vi "固件升级（包含参数恢复）.vi"() -> (3 "结果字符串":string)   [LabVIEW 2016, in "斯坦道总磷.lvlib"]
uses:
  <vilib>/NI/Progress Bar/Progress Bar.lvlib
  <vilib>/NI/Progress Bar/Controls/Progress Bar Properties.ctl
panel:
  out "固件升级步骤":T1
  # "固件升级步骤：\n1、读取固件状态\n2、读取仪器外设设置\n3、读取仪器试剂容量设置\n4、读取仪器量程参数设置\n5、读取仪器公式\n6、写入仪器固件\n7、写入仪器外设设置\n8、写入仪器试剂容量设置\n9、写入仪器量程参数设置\n10、写入仪器公式\n11、询问是否写入流程"
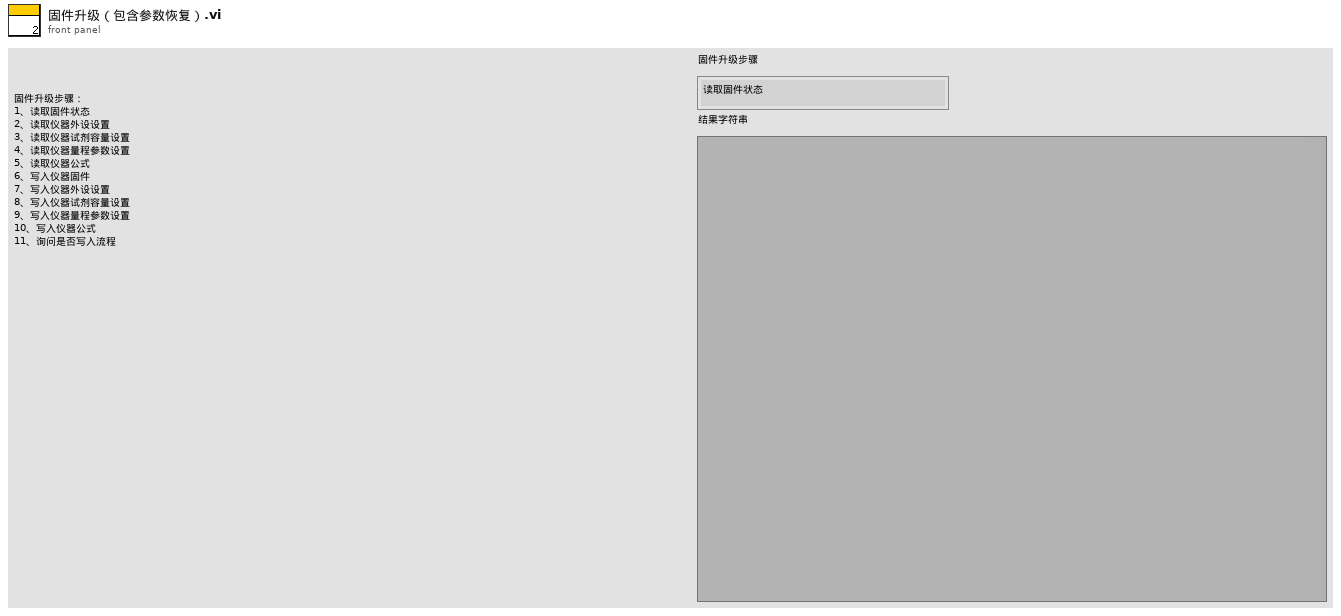
[diagram p1: front panel]
types:
  T1 = typedef "斯坦道总磷.lvlib/固件升级步骤.ctl" = enum16{"读取固件状态", "读取仪器外设设置", "读取仪器试剂容量设置", "读取仪器量程参数设置", "读取仪器公式", "写入仪器固件", "写入仪器外设设置", "写入仪器试剂容量设置", "写入仪器量程参数", "写入仪器公式", "询问是否写入流程", "写入测试流程", "结束"}
  T2 = typedef "Progress Bar.lvlib/Progress Bar Properties.ctl" = cluster{"Background Color":u32, "Installer Title":string, "Title Color":u32, "Action Text":string, "Text Color":u32, "Slider Value":u8, "Bar Color":u32, "Timeout":i32}
  T3 = cluster{"泵类型":u8, "进样速度":u32, "出样速度":u32, "泵阀量":u8, "光谱仪类型":u8, "光谱采样次数":u8, "氙灯次数":u8, "B":u16, "C":u16, "D":u16, "E":u16, "B_COD":u16, "C_COD":u16, "D_COD":u16, "E_COD":u16, "G":u16, "M":u16, "N":u16, "氨氮注射泵控温下限":sgl, "氨氮注射泵控温上限":sgl, "总氮注射泵控温下限":sgl, "总氮注射泵控温上限":sgl, "消解温度下限":sgl, "消解温度上限":sgl, "加热10s限值":sgl, "高温高压阀开阀温度":sgl, "总氮x公式0":u8, "总氮x公式1":sgl, "总氮x公式2":sgl, "总磷浊度稀释系数":sgl, "总磷浊度补偿权重1":sgl, "总磷浊度补偿权重2":sgl, "盐度系数":sgl, "氨氮补偿系数1":sgl, "氨氮补偿系数2":sgl}
  T4 = cluster{"外设配置":cluster{"泵类型":u8, "进样速度":u32, "出样速度":u32, "泵阀量":u8, "光谱仪类型":u8, "光谱采样次数":u8, "氙灯次数":u8, "B":u16, "C":u16, "D":u16, "E":u16, "B_COD":u16, "C_COD":u16, "D_COD":u16, "E_COD":u16, "G":u16, "M":u16, "N":u16, "氨氮注射泵控温下限":sgl, "氨氮注射泵控温上限":sgl, "总氮注射泵控温下限":sgl, "总氮注射泵控温上限":sgl, "消解温度下限":sgl, "消解温度上限":sgl, "加热10s限值":sgl, "高温高压阀开阀温度":sgl, "总氮x公式0":u8, "总氮x公式1":sgl, "总氮x公式2":sgl, "总磷浊度稀释系数":sgl, "总磷浊度补偿权重1":sgl, "总磷浊度补偿权重2":sgl, "盐度系数":sgl, "氨氮补偿系数1":sgl, "氨氮补偿系数2":sgl}, "error out":errorcluster}
  T5 = cluster{"V1":sgl, "V2":sgl, "V3":sgl, "V4":sgl, "V5":sgl, "V6":sgl, "V7":sgl, "V8":sgl, "V9":sgl, "V10":sgl, "V11":sgl, "V12":sgl, "V9-1":sgl, "V9-2":sgl}
  T6 = cluster{"试剂容量":cluster{"V1":sgl, "V2":sgl, "V3":sgl, "V4":sgl, "V5":sgl, "V6":sgl, "V7":sgl, "V8":sgl, "V9":sgl, "V10":sgl, "V11":sgl, "V12":sgl, "V9-1":sgl, "V9-2":sgl}, "error out":errorcluster}
  T7 = cluster{"测量精度":u16, "检出限":dbl, "上限":dbl, "下限":dbl, "阈值（低->高）":dbl, "阈值（高->低）":dbl, "稀释度":dbl}
  T8 = cluster{"Value":u16, "量程参数读取":cluster{"测量精度":u16, "检出限":dbl, "上限":dbl, "下限":dbl, "阈值（低->高）":dbl, "阈值（高->低）":dbl, "稀释度":dbl}, "error out":errorcluster}
  T9 = cluster{"Value":u16, i32, i32, "公式":cluster{"X^2":dbl, "X":dbl, "b":dbl}, "error out":errorcluster}
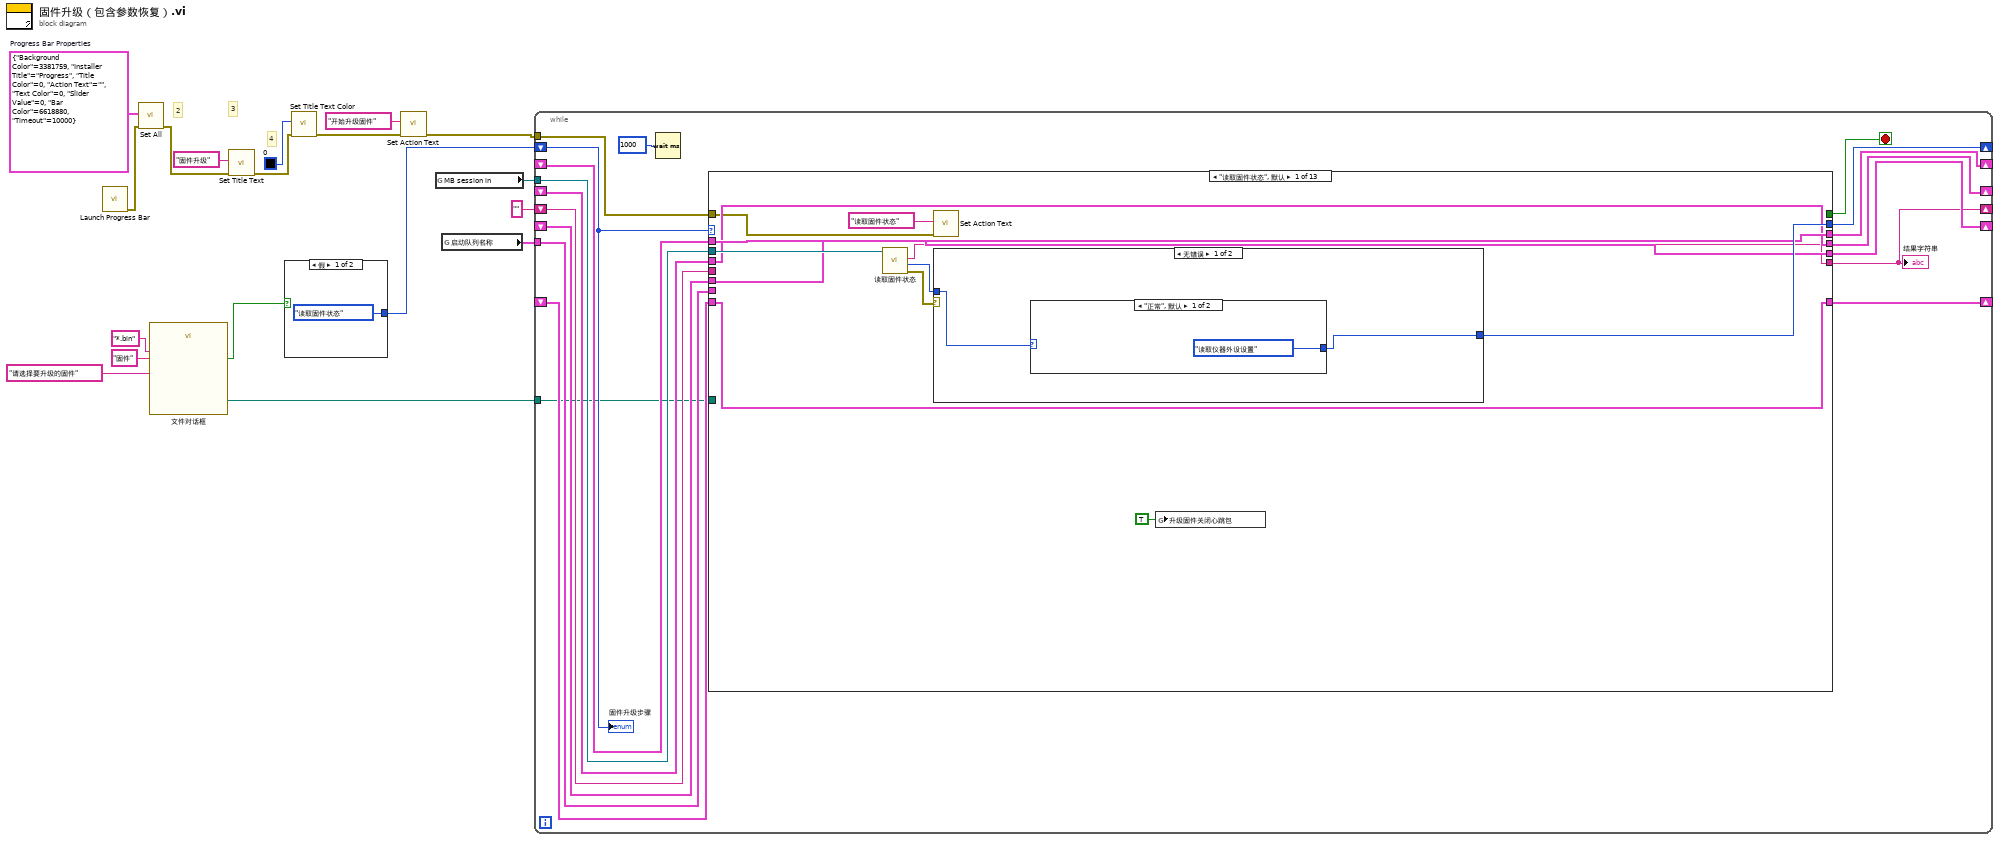
[diagram p0: block diagram]
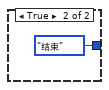
[diagram p2: hidden frame]
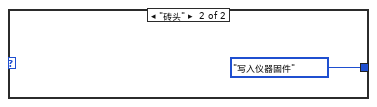
[diagram p3: hidden frame]
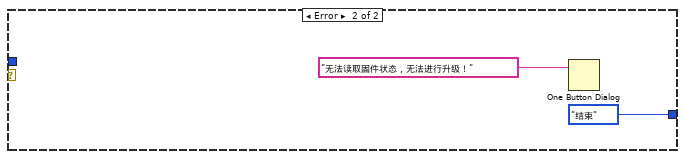
[diagram p4: hidden frame]
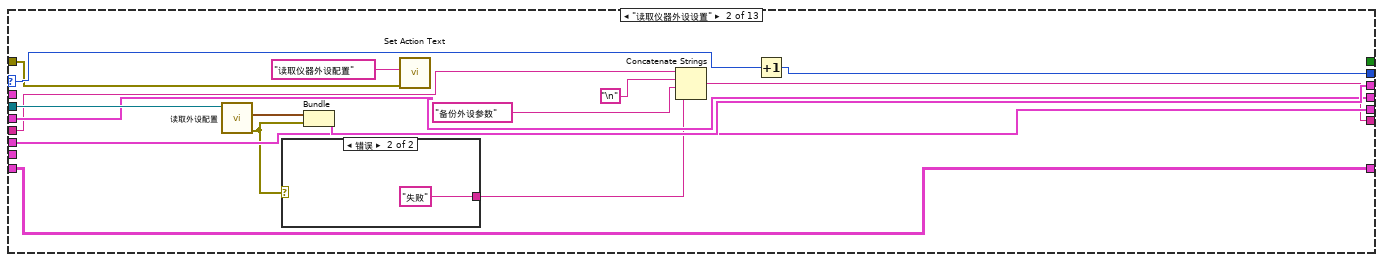
[diagram p5: hidden frame]
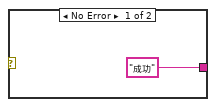
[diagram p6: hidden frame]
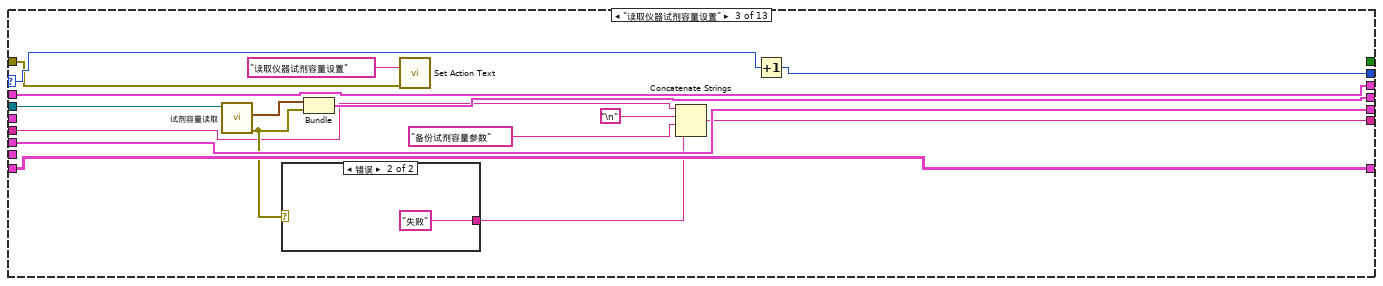
[diagram p7: hidden frame]
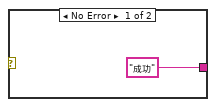
[diagram p8: hidden frame]
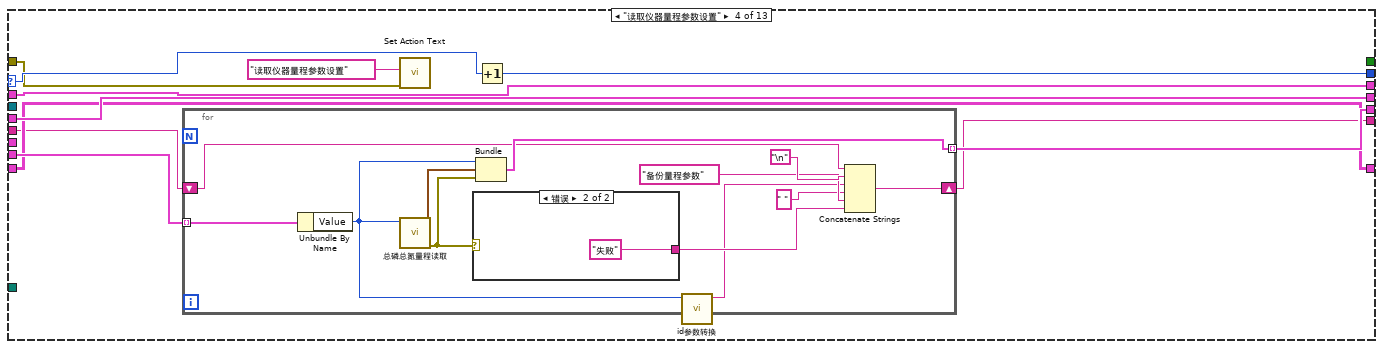
[diagram p9: hidden frame]
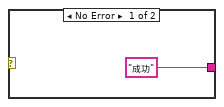
[diagram p10: hidden frame]
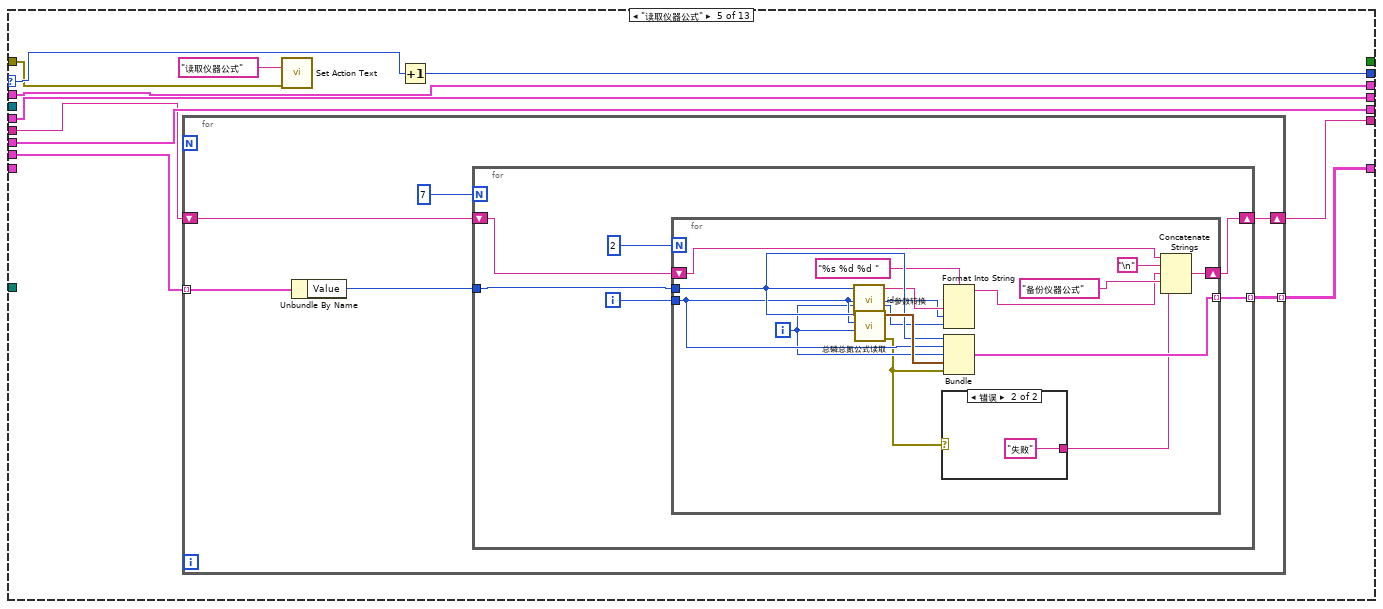
[diagram p11: hidden frame]
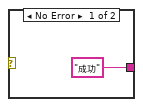
[diagram p12: hidden frame]
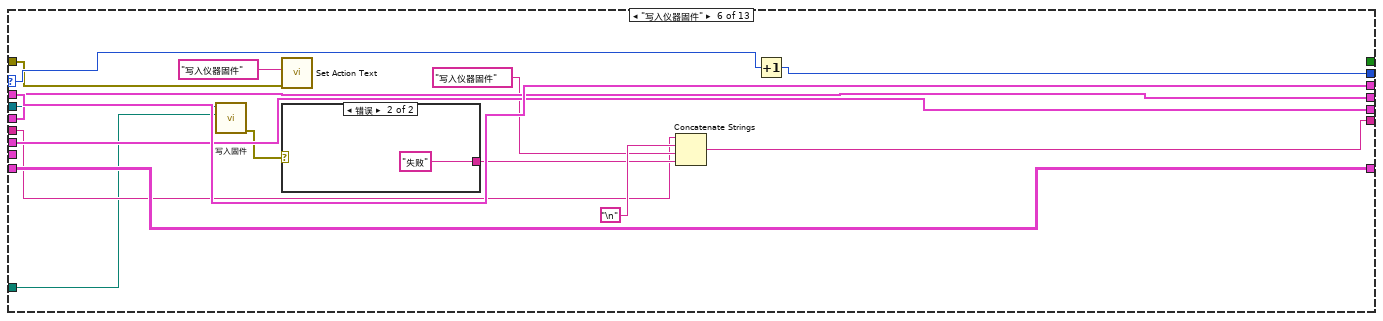
[diagram p13: hidden frame]
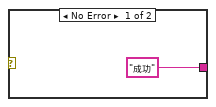
[diagram p14: hidden frame]
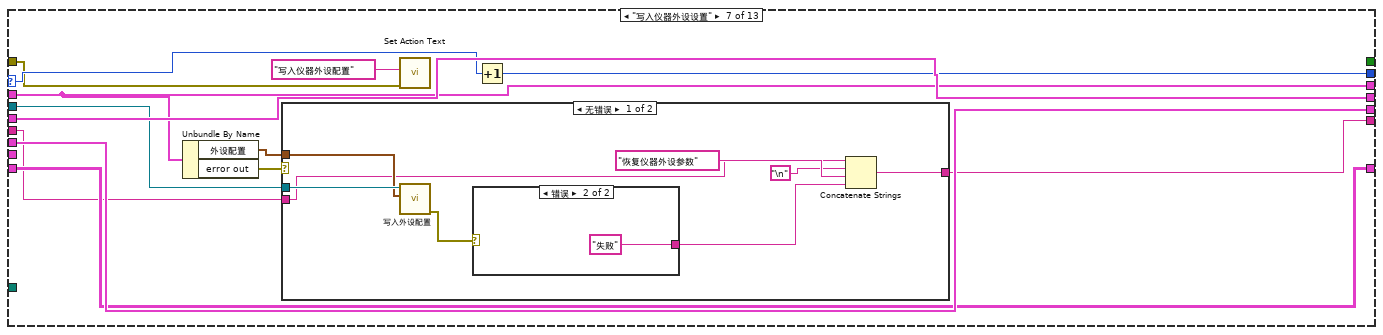
[diagram p15: hidden frame]
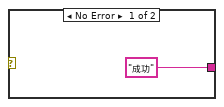
[diagram p16: hidden frame]
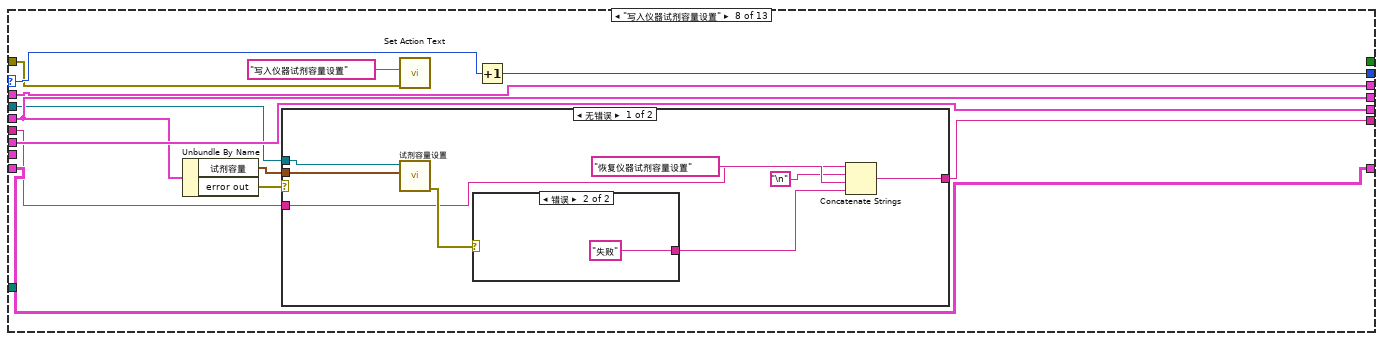
[diagram p18: hidden frame]
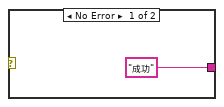
[diagram p19: hidden frame]
diagram:
  w15 = T2 {"Background Color"=3381759, "Installer Title"="Progress", "Title Color"=0, "Action Text"="", "Text Color"=0, "Slider Value"=0, "Bar Color"=6618880, "Timeout"=10000}  # Progress Bar Properties
  # "4"
  # "3"
  # "2"
  n1 = call <vilib>:"Launch Progress Bar.vi"() -> ("error out"=w14:errorcluster)  [unwired: 10 in, 1 out]
  n2 = call <vilib>:"Set All.vi"("error in (no error)"=w14, "Progress Bar Properties (Default)"=w15) -> ("error out"=w11:errorcluster)  [unwired: 9 in]
  n3 = call "文件对话框"("prompt"="请选择要升级的固件", "pattern (all files)"="*.bin", "pattern label"="固件") -> ("selected path"=w3:path, "cancelled"=w2:bool)  [unwired: 9 in, 2 out]
  n4 = call <vilib>:"Set Title Text.vi"("error in (no error)"=w11, "Installer Title"="固件升级") -> ("error out"=w9:errorcluster)  [unwired: 9 in]
  n5 = case shown="假" w2 {
    tunnel: [固件升级步骤."读取固件状态" ("固件升级步骤") 固件升级步骤."结束" ("固件升级步骤")] -> w1
    frame False {
    }
    frame True {
    }
  }
  n6 = call <vilib>:"Set Title Text Color.vi"("error in (no error)"=w9, "Color Box"=u32 0) -> ("error out"=w12:errorcluster)  [unwired: 9 in]
  n7 = call <vilib>:"Set Action Text.vi"("error in (no error)"=w12, "Action Text"="开始升级固件") -> ("error out"=w7:errorcluster)  [unwired: 9 in]
  n8 = global read "VAR总磷总氮全局变量.vi" "MB session in"() -> (w18:refnum<class "MB_Master.lvclass">)
  n9 = global read "总磷总氮断电保存全局变量.vi" "启动队列名称"() -> (w17:cluster{"String":string, "Value":u16}[])
  n10 = while {
    tunnel: w18 -> [w37]
    shift-right: [w36] -> _
    shift-left: w1 -> [w38]
    shift-right: [w34] -> _
    shift-left: _ -> [w33]
    shift-right: [w32] -> _
    shift-left: _ -> [w31]
    tunnel: w17 -> [w30]
    shift-right: [w29] -> _
    shift-left: _ -> [w28]
    shift-right: [w27] -> _
    shift-left: _ -> [w26]
    shift-right: [w23] -> _
    shift-left: "" ("结果字符串") -> [w24]
    tunnel: w7 -> [w22]
    tunnel: w3 -> [w21]
    stop <- w35 stop-if-true
    n11 = Wait (ms)(milliseconds to wait=u32 1000 ("等待时间（毫秒）")) -> ()  [unwired: 1 out]
    n12 = case shown="\"读取固件状态\", 默认" w38 {
      selector: w38 -> [_ w69 w87 w98 w123 w167 w181 w208 w230 w259 w294 w309 w326]
      tunnel: w37 -> [w50 w72 w90 _ _ w168 w184 w204 _ _ _ _ _]
      tunnel: [w47 w68 w86 w97 w122 w166 w180 w207 w229 w258 w293 w308 w326] -> w36
      tunnel: [_ _ _ _ _ _ _ _ _ _ _ _ TRUE] -> w35
      tunnel: [w46 w70 w85 w101 w126 w172 w183 w211 w232 w261 w300 w315 w325] -> w34
      tunnel: w33 -> [w46 _ w85 w101 w126 w172 w183 w211 w232 w261 w300 w315 w325]
      tunnel: [w45 w67 w88 w100 w125 w171 w187 w206 w228 w260 w299 w314 w324] -> w32
      tunnel: w31 -> [w45 w67 _ w100 w125 w171 w187 w206 w228 w260 w299 w314 w324]
      tunnel: w30 -> [_ _ _ w103 w128 _ _ _ _ _ _ _ _]
      tunnel: [w44 w66 w84 w102 w124 w170 w186 w210 w227 w257 w298 w313 w323] -> w29
      tunnel: w28 -> [w44 w66 w84 _ w124 w170 w186 w210 w227 w257 w298 w313 w323]
      tunnel: [w43 w65 w83 w99 w127 w169 w185 w209 w231 w256 w297 w312 w322] -> w27
      tunnel: w26 -> [w43 w65 w83 w99 _ w169 w185 w209 w231 w256 w297 w312 w322]
      tunnel: [w42 w63 w77 w95 w120 w161 w178 w201 w225 w254 w292 w306 w318] -> w23
      tunnel: w24 -> [_ w62 w78 w96 w121 w162 w177 w202 w226 w255 w292 w307 w319]
      tunnel: w22 -> [w41 w57 w75 w93 w118 w158 w175 w199 w223 w252 _ _ w317]
      tunnel: w21 -> [_ _ _ _ _ w157 _ _ _ _ _ _ _]
      frame "读取固件状态", Default {
        n13 = call "读取固件状态.vi"("MB session in"=w50) -> ("error out"=w48:errorcluster, "固件状态"=w49:enum16{"正常", "砖头"}, "结果字符串"=w42:string)  [unwired: 7 in, 1 out]
        n14 = call <vilib>:"Set Action Text.vi"("error in (no error)"=w41, "Action Text"="读取固件状态") -> ()  [unwired: 9 in, 1 out]
        n15 = case shown="无错误" w48 {
          tunnel: w49 -> [w52 _]
          tunnel: [w51 固件升级步骤."结束" ("固件升级步骤")] -> w47
          frame No Error {
            n16 = case shown="\"正常\", 默认" w52 {
              tunnel: [固件升级步骤."读取仪器外设设置" ("固件升级步骤") 固件升级步骤."写入仪器固件" ("固件升级步骤")] -> w51
              frame "正常", Default {
              }
              frame "砖头" {
              }
            }
          }
          frame Error {
            n17 = One Button Dialog(message="无法读取固件状态，无法进行升级！" ("消息")) -> ()  [unwired: 1 in, 1 out]
          }
        }
        n18 = global write "VAR总磷总氮全局变量.vi" "升级固件关闭心跳包"(TRUE ("升级固件关闭心跳包")) -> ()
      }
      frame "读取仪器外设设置" {
        n19 = call "读取外设配置.vi"("MB session in"=w72) -> ("error out"=w64:errorcluster, "外设配置"=w71:T3)  [unwired: 8 in, 1 out]
        n20 = case shown="错误" w64 {
          tunnel: ["成功" "失败"] -> w60
          frame No Error {
          }
          frame Error {
          }
        }
        n21 = Bundle("外设配置"=w71, "error out"=w64) -> (w70:T4)  [unwired: 1 in]
        n22 = call <vilib>:"Set Action Text.vi"("error in (no error)"=w57, "Action Text"="读取仪器外设配置") -> ()  [unwired: 9 in, 1 out]
        n23 = Concatenate Strings(w62, "\n", "备份外设参数" ("字符串"), w60) -> (w63:string)
        n24 = Increment(x=w69) -> (x+1=w68:T1)
      }
      frame "读取仪器试剂容量设置" {
        n25 = call "试剂容量读取.vi"("MB session in"=w90) -> ("error out"=w79:errorcluster, "试剂容量"=w89:T5)  [unwired: 8 in, 1 out]
        n26 = case shown="错误" w79 {
          tunnel: ["成功" "失败"] -> w81
          frame No Error {
          }
          frame Error {
          }
        }
        n27 = Bundle("试剂容量"=w89, "error out"=w79) -> (w88:T6)  [unwired: 1 in]
        n28 = call <vilib>:"Set Action Text.vi"("error in (no error)"=w75, "Action Text"="读取仪器试剂容量设置") -> ()  [unwired: 9 in, 1 out]
        n29 = Concatenate Strings(w78, "\n", "备份试剂容量参数" ("字符串"), w81) -> (w77:string)
        n30 = Increment(x=w87) -> (x+1=w86:T1)
      }
      frame "读取仪器量程参数设置" {
        n31 = for {
          tunnel: w103 -> [w115] mode=indexing
          tunnel: [w113] -> w102 mode=indexing
          shift-right: [w107] -> w95
          shift-left: w96 -> [w108]
          n32 = Unbundle By Name(w115) -> ("Value"=w106:u16)
          n33 = call "总磷总氮量程读取.vi"("测量参数"=w106) -> ("error out"=w109:errorcluster, "量程参数读取"=w114:T7)  [unwired: 9 in]
          n34 = case shown="错误" w109 {
            tunnel: ["成功" "失败"] -> w111
            frame No Error {
            }
            frame Error {
            }
          }
          n35 = Bundle("Value"=w106, "量程参数读取"=w114, "error out"=w109) -> (w113:T8)  [unwired: 1 in]
          n36 = call "id参数转换.vi"("id"=w106) -> ("table输出"=w105:string)  [unwired: 9 in, 1 out]
          n37 = Concatenate Strings(w108, "\n", w105, " " ("字符串"), "备份量程参数" ("字符串"), w111) -> (w107:string)
        }
        n38 = call <vilib>:"Set Action Text.vi"("error in (no error)"=w93, "Action Text"="读取仪器量程参数设置") -> ()  [unwired: 9 in, 1 out]
        n39 = Increment(x=w98) -> (x+1=w97:T1)
      }
      frame "读取仪器公式" {
        n40 = for {
          tunnel: w128 -> [w134] mode=indexing
          tunnel: [w131] -> w127 mode=indexing
          shift-right: [w129] -> w120
          shift-left: w121 -> [w130]
          n41 = Unbundle By Name(w134) -> ("Value"=w132:u16)
          n42 = for {
            N: 7 -> [_]
            tunnel: w132 -> [w140]
            tunnel: [w137] -> w131 mode=indexing
            shift-right: [w136] -> w129
            shift-left: w130 -> [w135]
            i -> [w139]
            n43 = for {
              N: 2 -> [_]
              tunnel: w140 -> [w147]
              tunnel: w139 -> [w144]
              tunnel: [w153] -> w137 mode=indexing
              shift-right: [w149] -> w136
              shift-left: w135 -> [w148]
              i -> [w143]
              n44 = call "id参数转换.vi"("id"=w147) -> ("table输出"=w145:string)  [unwired: 9 in, 1 out]
              n45 = call "总磷总氮公式读取.vi"("量程"=w143, "测量模式"=w144, "测量参数"=w147) -> ("error out"=w141:errorcluster, "公式"=w154:cluster{"X^2":dbl, "X":dbl, "b":dbl})  [unwired: 7 in]
              n46 = case shown="错误" w141 {
                tunnel: ["成功" "失败"] -> w151
                frame No Error {
                }
                frame Error {
                }
              }
              n47 = Format Into String(format string="%s %d %d " ("格式字符串"), w145, w144, w143) -> (resulting string=w142:string)  [unwired: 2 in, 1 out]
              n48 = Bundle("Value"=w147, w144, w143, "公式"=w154, "error out"=w141) -> (w153:T9)  [unwired: 1 in]
              n49 = Concatenate Strings(w148, "\n", w142, "备份仪器公式" ("字符串"), w151) -> (w149:string)
            }
          }
        }
        n50 = call <vilib>:"Set Action Text.vi"("error in (no error)"=w118, "Action Text"="读取仪器公式") -> ()  [unwired: 9 in, 1 out]
        n51 = Increment(x=w123) -> (x+1=w122:T1)
      }
      frame "写入仪器固件" {
        n52 = call "写入固件.vi"("selected path"=w157, "MB session in"=w168) -> ("error out"=w160:errorcluster)  [unwired: 8 in, 1 out]
        n53 = call <vilib>:"Set Action Text.vi"("error in (no error)"=w158, "Action Text"="写入仪器固件") -> ()  [unwired: 9 in, 1 out]
        n54 = case shown="错误" w160 {
          tunnel: ["成功" "失败"] -> w164
          frame No Error {
          }
          frame Error {
          }
        }
        n55 = Concatenate Strings(w162, "\n", "写入仪器固件" ("字符串"), w164) -> (w161:string)
        n56 = Increment(x=w167) -> (x+1=w166:T1)
      }
      frame "写入仪器外设设置" {
        n57 = Unbundle By Name(w183) -> ("外设配置"=w182:T3, "error out"=w179:errorcluster)
        n58 = case shown="无错误" w179 {
          tunnel: w184 -> [w195 _]
          tunnel: w182 -> [w194 _]
          tunnel: [w189 w198] -> w178
          tunnel: w177 -> [w188 w198]
          frame No Error {
            n59 = call "写入外设配置.vi"("外设配置"=w194, "MB session in"=w195) -> ("error out"=w190:errorcluster)  [unwired: 8 in, 1 out]
            n60 = case shown="错误" w190 {
              tunnel: ["成功" "失败"] -> w192
              frame No Error {
              }
              frame Error {
              }
            }
            n61 = Concatenate Strings(w188, "\n", "恢复仪器外设参数" ("字符串"), w192) -> (w189:string)
          }
          frame Error {
          }
        }
        n62 = call <vilib>:"Set Action Text.vi"("error in (no error)"=w175, "Action Text"="写入仪器外设配置") -> ()  [unwired: 9 in, 1 out]
        n63 = Increment(x=w181) -> (x+1=w180:T1)
      }
      frame "写入仪器试剂容量设置" {
        n64 = Unbundle By Name(w206) -> ("试剂容量"=w205:T5, "error out"=w203:errorcluster)
        n65 = case shown="无错误" w203 {
          tunnel: w205 -> [w219 _]
          tunnel: w204 -> [w218 _]
          tunnel: w202 -> [w213 w222]
          tunnel: [w212 w222] -> w201
          frame No Error {
            n66 = call "试剂容量设置.vi"("试剂容量"=w219, "MB session in"=w218) -> ("error out"=w214:errorcluster)  [unwired: 8 in, 1 out]
            n67 = case shown="错误" w214 {
              tunnel: ["成功" "失败"] -> w216
              frame No Error {
              }
              frame Error {
              }
            }
            n68 = Concatenate Strings(w213, "\n", "恢复仪器试剂容量设置" ("字符串"), w216) -> (w212:string)
          }
          frame Error {
          }
        }
        n69 = call <vilib>:"Set Action Text.vi"("error in (no error)"=w199, "Action Text"="写入仪器试剂容量设置") -> ()  [unwired: 9 in, 1 out]
        n70 = Increment(x=w208) -> (x+1=w207:T1)
      }
      frame "写入仪器量程参数" {
        n71 = for {
          tunnel: w227 -> [w238] mode=indexing
          shift-right: [w233] -> w225
          shift-left: w226 -> [w234]
          n72 = Unbundle By Name(w238) -> ("Value"=w236:u16, "量程参数读取"=w237:T7, "error out"=w235:errorcluster)
          n73 = case shown="无错误" w235 {
            tunnel: w237 -> [w248 _]
            tunnel: w236 -> [w241 _]
            tunnel: w234 -> [w243 w251]
            tunnel: [w242 w251] -> w233
            frame No Error {
              n74 = call "总磷总氮量程写入.vi"("量程参数写入"=w248, "测量参数"=w241) -> ("error out"=w244:errorcluster)  [unwired: 8 in]
              n75 = case shown="无错误" w244 {
                tunnel: ["成功" "失败"] -> w246
                frame No Error {
                }
                frame Error {
                }
              }
              n76 = call "id参数转换.vi"("id"=w241) -> ("table输出"=w240:string)  [unwired: 9 in, 1 out]
              n77 = Concatenate Strings(w243, "\n", w240, " " ("字符串"), "恢复仪器量程参数" ("字符串"), w246) -> (w242:string)
            }
            frame Error {
            }
          }
        }
        n78 = call <vilib>:"Set Action Text.vi"("error in (no error)"=w223, "Action Text"="写入仪器量程参数设置") -> ()  [unwired: 9 in, 1 out]
        n79 = Increment(x=w230) -> (x+1=w229:T1)
      }
      frame "写入仪器公式" {
        n80 = for {
          tunnel: w256 -> [w264] mode=indexing
          shift-right: [w262] -> w254
          shift-left: w255 -> [w263]
          n81 = for {
            tunnel: w264 -> [w267] mode=indexing
            shift-right: [w265] -> w262
            shift-left: w263 -> [w266]
            n82 = for {
              tunnel: w267 -> [w275] mode=indexing
              shift-right: [w268] -> w265
              shift-left: w266 -> [w269]
              n83 = Unbundle(w275) -> ("Value"=w273:u16, w272:i32, w271:i32, "公式"=w270:cluster{"X^2":dbl, "X":dbl, "b":dbl}, "error out"=w274:errorcluster)
              n84 = case shown="无错误" w274 {
                tunnel: w273 -> [w280 _]
                tunnel: w272 -> [w279 _]
                tunnel: w271 -> [w278 _]
                tunnel: w270 -> [w288 _]
                tunnel: w269 -> [w277 w291]
                tunnel: [w276 w291] -> w268
                frame No Error {
                  n85 = call "总磷总氮公式写入.vi"("公式"=w288, "量程"=w278, "测量模式"=w279, "测量参数"=w280) -> ("error out"=w281:errorcluster)  [unwired: 7 in]
                  n86 = case shown="错误" w281 {
                    tunnel: ["成功" "失败"] -> w286
                    frame No Error {
                    }
                    frame Error {
                    }
                  }
                  n87 = call "id参数转换.vi"("id"=w280) -> ("table输出"=w283:string)  [unwired: 9 in, 1 out]
                  n88 = Format Into String(format string="%s %d %d " ("格式字符串"), w283, w279, w278) -> (resulting string=w282:string)  [unwired: 2 in, 1 out]
                  n89 = Concatenate Strings(w277, "\n", w282, "恢复仪器公式" ("字符串"), w286) -> (w276:string)
                }
                frame Error {
                }
              }
            }
          }
        }
        n90 = call <vilib>:"Set Action Text.vi"("error in (no error)"=w252, "Action Text"="写入仪器公式") -> ()  [unwired: 9 in, 1 out]
        n91 = Increment(x=w259) -> (x+1=w258:T1)
      }
      frame "询问是否写入流程" {
        n92 = Two Button Dialog(message="是否写入流程" ("消息")) -> (T button?=w295:bool)  [unwired: 2 in]
        n93 = case shown="假" w295 {
          tunnel: w294 -> [_ w303]
          tunnel: [固件升级步骤."结束" w302] -> w293
          frame False {
          }
          frame True {
            n94 = Increment(x=w303) -> (x+1=w302:T1)
          }
        }
      }
      frame "写入测试流程" {
        n95 = Concatenate Strings(w307, "\n", "写入流程" ("字符串")) -> (w306:string)
        n96 = global read "总磷总氮断电保存全局变量.vi" "简易流程路径"() -> (w310:path)
        n97 = global read "总磷总氮断电保存全局变量.vi" "流程路径"() -> (w311:path)
        n98 = call "流程写入.vi"("简易流程路径"=w310, "添加的路径"=w311) -> ()  [unwired: 10 in]
        n99 = Increment(x=w309) -> (x+1=w308:T1)
      }
      frame "结束" {
        n100 = call <vilib>:"Close Progress Bar.vi"("error in (no error)"=w317) -> ()  [unwired: 9 in, 2 out]
        n101 = Concatenate Strings(w319, "\n", "结束" ("字符串")) -> (w318:string)
        n102 = global write "VAR总磷总氮全局变量.vi" "升级固件关闭心跳包"(FALSE ("升级固件关闭心跳包")) -> ()
      }
    }
    "结果字符串" <- w23
    "固件升级步骤" <- w38
  }
